vi "CP0dll.vi"(8 "error in (no error)":errorcluster, 9 "Cp":dbl, 10 "z":dbl[](array[numeric]), 11 "t":dbl) -> (0 "error out":errorcluster, 1 "Cp out":dbl, 2 "z out":dbl[](array[numeric]), 3 "t out":dbl)   [LabVIEW 2016]
doc: "subroutine CP0dll(t, z, cp)\n\nCalculate Cp0 for a mixture given temperature and composition.\n\nINPUTS:\nt -- Temperature [K]\nz -- Composition array (array of mole fractions)\n\nOUTPUTS:\ncp--isobaric (constant p) heat capacity [J/mol-K]"
uses:
  REFPROP.DLL
panel:
  # "REFPROP-CP0dll.vi"
  # "void  CP0dll(double *t, double *z, double *Cp);"
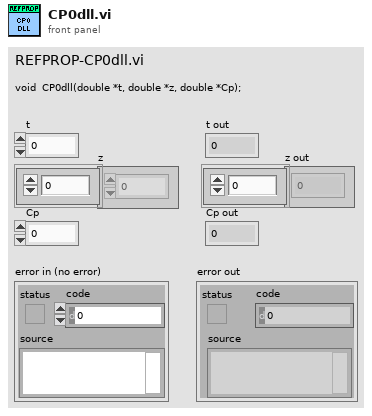
[diagram p1: front panel]
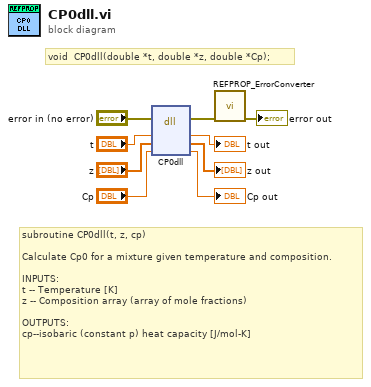
[diagram p0: block diagram]
diagram:
  # "void  CP0dll(double *t, double *z, double *Cp);"
  # "subroutine CP0dll(t, z, cp)\n\nCalculate Cp0 for a mixture given temperature and composition.\n\nINPUTS:\nt -- Temperature [K]\nz -- Composition array (array of mole fractions)\n\nOUTPUTS:\ncp--isobaric (constant p) heat capacity [J/mol-K]"
  n1 = dll-call lib="S:/009 - Testing/02 - Performance Testing/REFPROP/REFPROP.*" fn="CP0dll"(error in="error in (no error)", "t"="t", "z"="z", "Cp"="Cp") -> (error out=w3:errorcluster, "t"=→"t out":dbl, "z"=→"z out":dbl[], "Cp"=→"Cp out":dbl)  [unwired: 3 in, 1 out]
  n2 = call "REFPROP_ErrorConverter.vi"("error in (no error)"=w3) -> ("error out"=→"error out":errorcluster)  [unwired: 10 in]
